vi "QueueManagerGV.vi"(7 "Command":enum16{"Get", "Set"}(ring), 11 "Queue in":refnum<queue>) -> (3 "Queue":refnum<queue>)   [LabVIEW 2014]
uses:
  Type Defs/telemetryReading.ctl
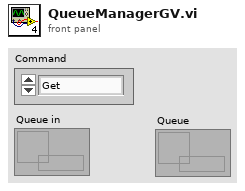
[diagram p1: front panel]
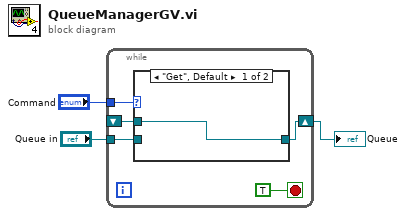
[diagram p0: block diagram]
diagram:
  n1 = while {
    tunnel: "Command" -> [w8]
    tunnel: "Queue in" -> [w5]
    shift-right: [w6] -> w1
    shift-left: _ -> [w4]
    stop <- TRUE stop-if-true
    n2 = case shown="\"Get\", Default" w8 {
      tunnel: [w9 w10] -> w6
      tunnel: w5 -> [_ w10]
      tunnel: w4 -> [w9 _]
      frame "Get", Default {
      }
      frame "Set" {
      }
    }
  }
  "Queue" <- w1
